vi "initGcode.vi"(6 "Che Do":bool=TRUE, 7 "gCode":T1, 8 "error in (no error)":errorcluster, 9 "PosSetG92":cluster{"X":dbl, "Y":dbl, "Z":dbl}, 10 "Gcode In":string, 11 "XuLyDataDisplay in":refnum<class "XuLyDataDisplay.lvclass">) -> (0 "error out":errorcluster, 2 "GcodeString Out":string, 3 "XuLyDataDisplay out":refnum<class "XuLyDataDisplay.lvclass">)   [LabVIEW 2017, in "LibraryGcode.lvlib" / "XuLyDataDisplay.lvclass"]
uses:
  XuLyDataDisplay.lvclass
  SelectGcode.ctl
  01552a10-2ba1-4855-bc3a-b1e10501afc1.vi
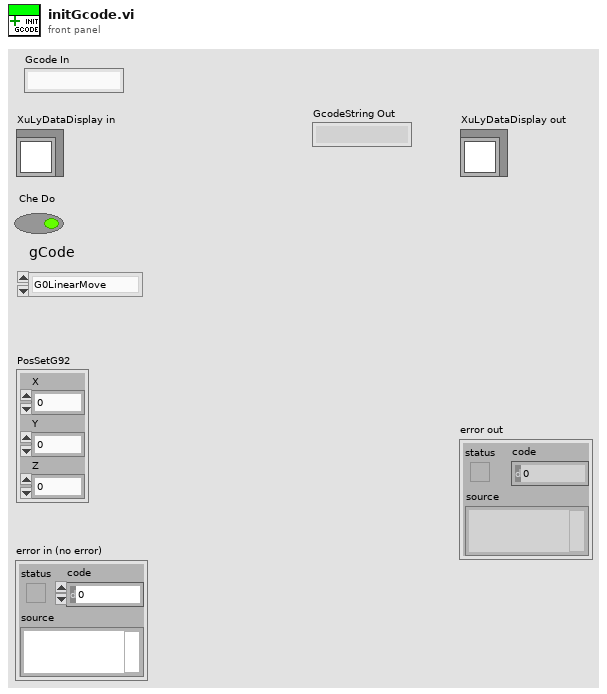
[diagram p1: front panel]
types:
  T1 = typedef "LibraryGcode.lvlib/XuLyDataDisplay.lvclass/SelectGcode.ctl" = enum16{"G0LinearMove", "G1XY", "G1LinearMove", "G2Arc", "G4Dwell", "G20InchUnit", "G21MilliUnit", "G28AutoHome", "G92SetPosition", "G90", "G91RelativePos", "JogX+", "JogX-", "JogY+", "JogY-", "JogZ+", "JogZ-", "sendGcodeString"}
  T2 = enum16{"Fan1", "Fan2", "Fan3", "PARA", "POS_DEGREE", "Solenoid", "Spindle", "TypeFirmware", "WaitPin", "MaxAcel", "MaxFeedrate", "MaxSize", "MaxStartAccel"}
  T3 = typedef "LibraryGcode.lvlib/TypeFirmwareControl.ctl" = enum16{"ScaraMarlin", "CncMarlin", "Mk4Due"}
  T4 = cluster{"PWM":dbl, "TypeFirmware":T3, "XYZ":cluster{"X":dbl, "Y":dbl, "Z":dbl}, "PARA":cluster{"STEP":i16, "FEEDRATE":dbl}, "DEGREES":cluster{"X":dbl, "Y":dbl}, "Solenoid":bool, "StartAccel":cluster{"P":dbl, "R":dbl, "T":dbl}}
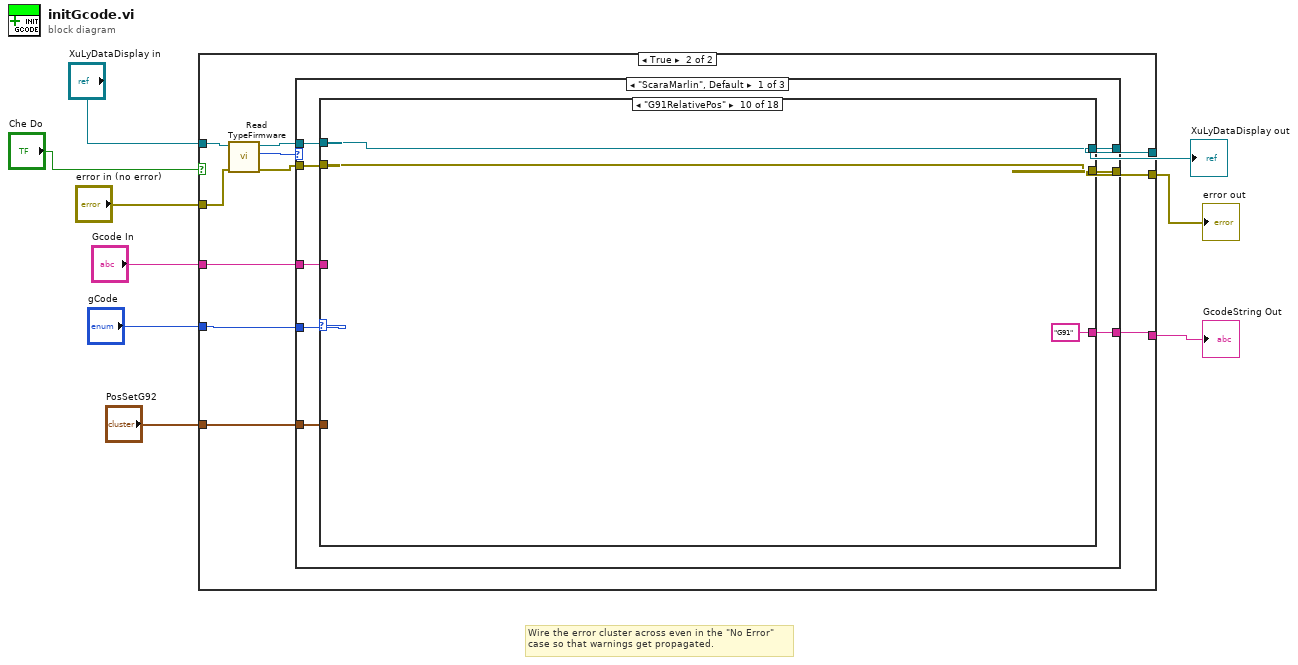
[diagram p0: block diagram]
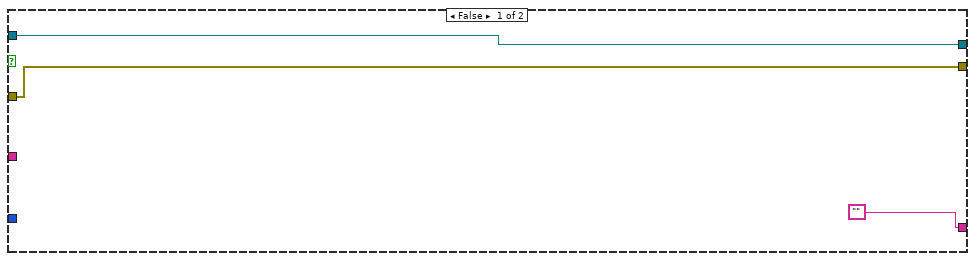
[diagram p2: hidden frame]
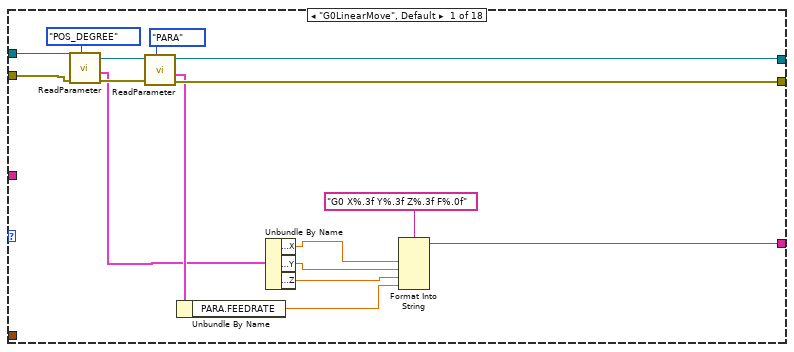
[diagram p3: hidden frame]
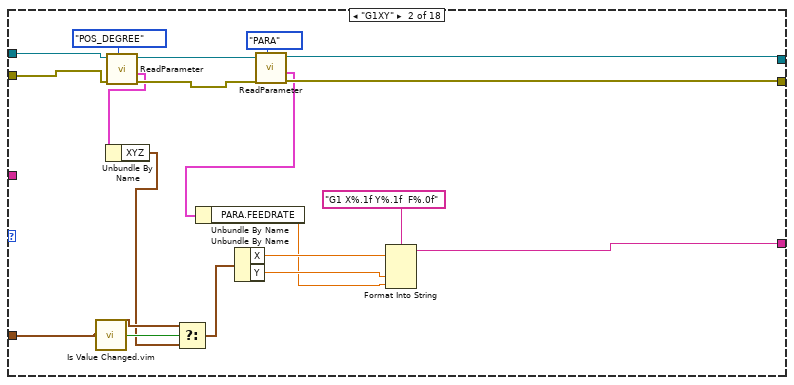
[diagram p4: hidden frame]
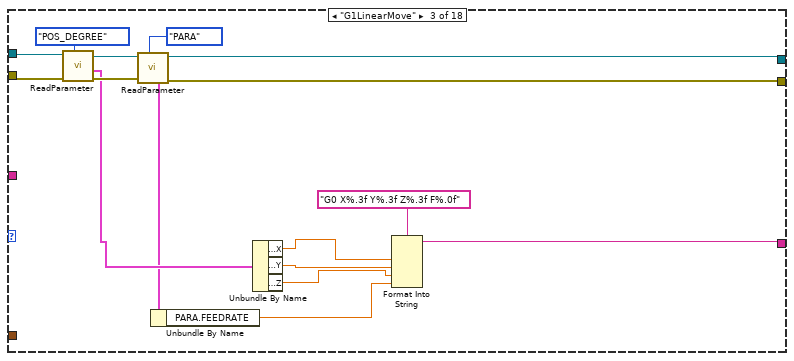
[diagram p5: hidden frame]
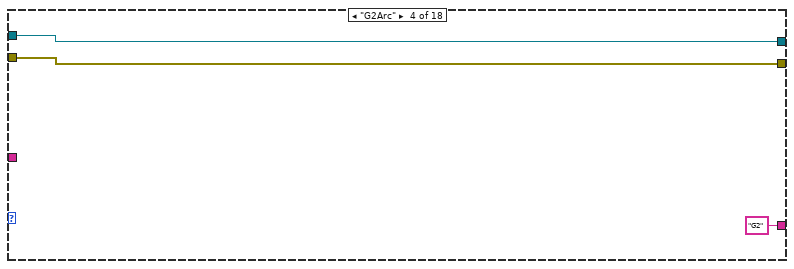
[diagram p6: hidden frame]
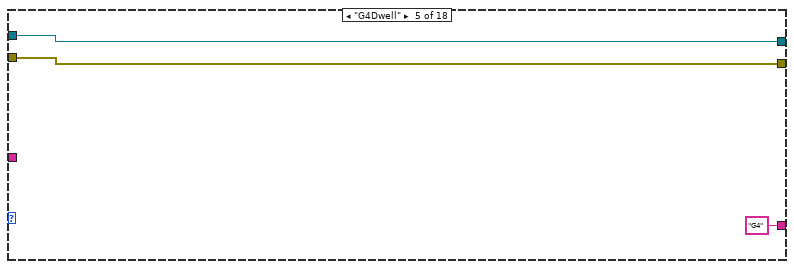
[diagram p7: hidden frame]
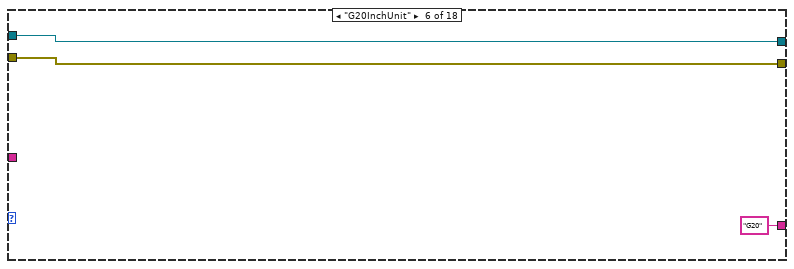
[diagram p8: hidden frame]
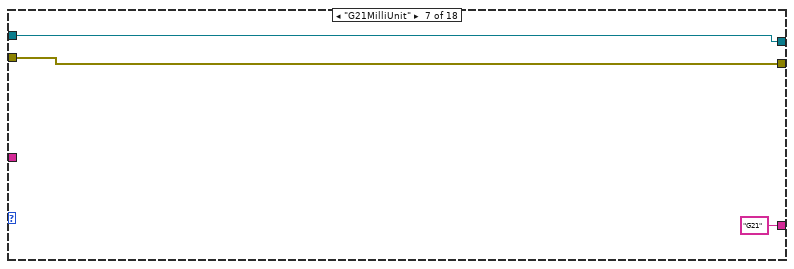
[diagram p9: hidden frame]
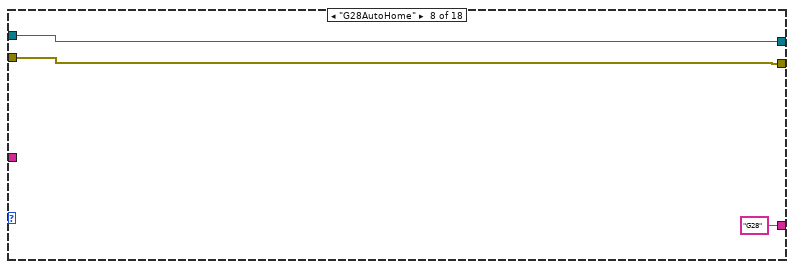
[diagram p10: hidden frame]
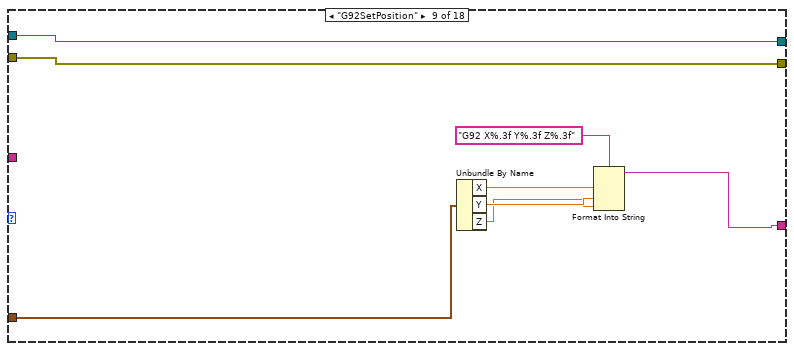
[diagram p11: hidden frame]
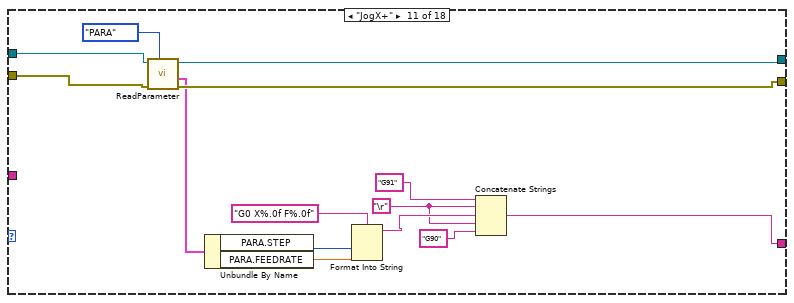
[diagram p12: hidden frame]
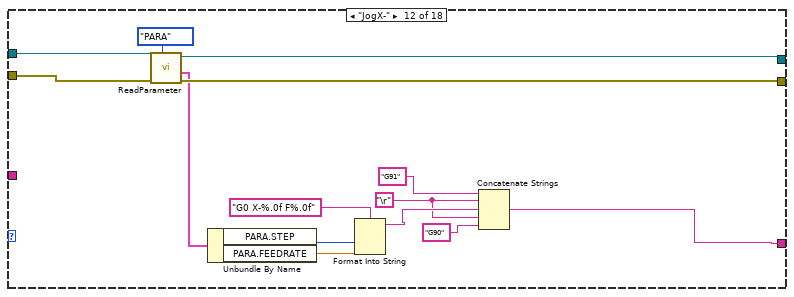
[diagram p13: hidden frame]
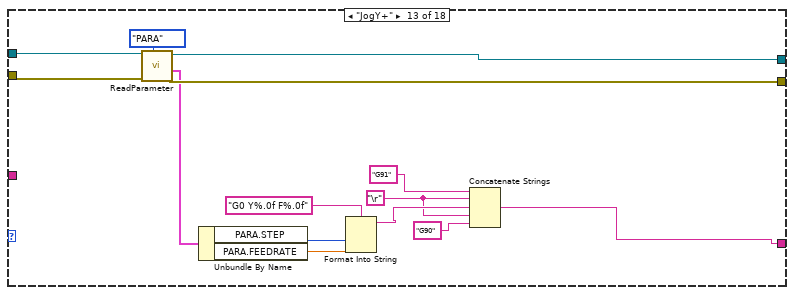
[diagram p14: hidden frame]
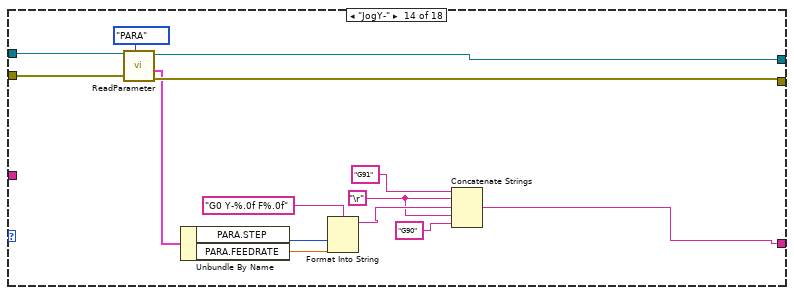
[diagram p15: hidden frame]
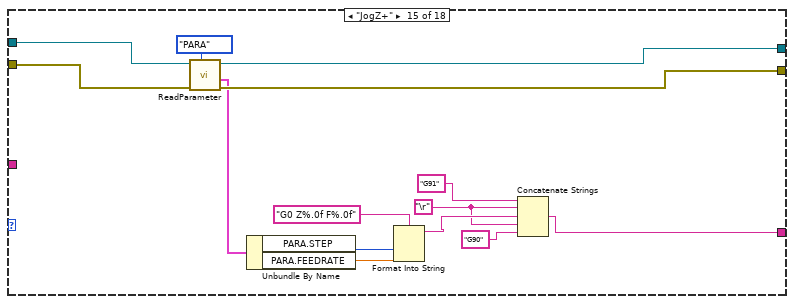
[diagram p16: hidden frame]
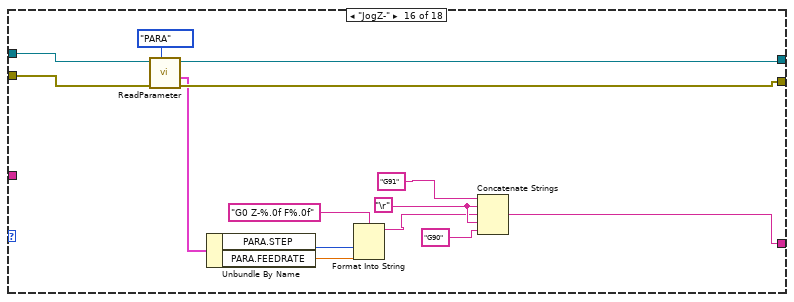
[diagram p17: hidden frame]
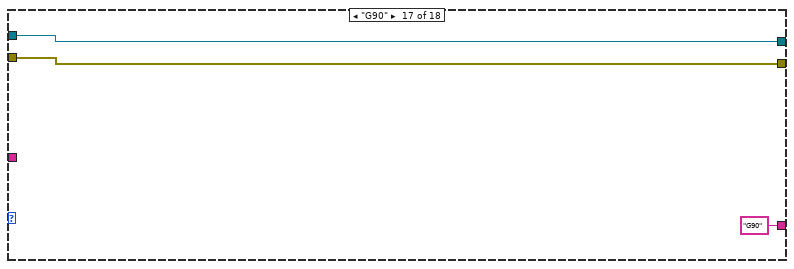
[diagram p18: hidden frame]
diagram:
  # "Wire the error cluster across even in the \"No Error\"\ncase so that warnings get propagated."
  n1 = case shown="True" "Che Do" {
    tunnel: [w11 w18] -> w9
    tunnel: [w12 w23] -> w8
    tunnel: "XuLyDataDisplay in" -> [w12 w21]
    tunnel: "gCode" -> [_ w17]
    tunnel: ["" w13] -> w5
    tunnel: "PosSetG92" -> [_ w16]
    tunnel: "error in (no error)" -> [w11 w15]
    tunnel: "Gcode In" -> [_ w14]
    frame False {
    }
    frame True {
      n2 = call-dynamic "Read TypeFirmware.vi"("error in (no error)"=w15, "ParameterConf in"=w21) -> ("error out"=w19:errorcluster, "TypeFirmware"=w20:T3, "ParameterConf out"=w22:refnum<class "XuLyDataDisplay.lvclass">)  [unwired: 7 in]
      n3 = case shown="\"ScaraMarlin\", Default" w20 {
        tunnel: [w28 w203 w209] -> w23
        tunnel: w22 -> [w27 w202 w209]
        tunnel: w19 -> [w29 w200 w208]
        tunnel: [w30 w201 w208] -> w18
        tunnel: w17 -> [w31 w199 _]
        tunnel: w16 -> [w26 _ _]
        tunnel: w14 -> [w24 _ _]
        tunnel: [w25 _ _] -> w13
        frame "ScaraMarlin", Default {
          n4 = case shown="\"G91RelativePos\"" w31 {
            tunnel: [w38 w59 w73 w83 w86 w89 w92 w95 w98 w106 w112 w126 w141 w154 w169 w181 w193 w196] -> w30
            tunnel: w29 -> [w40 w55 w74 w83 w86 w89 w92 w95 w98 w106 w114 w128 w140 w156 w168 w186 w193 w196]
            tunnel: [w37 w60 w72 w84 w87 w90 w93 w96 w99 w107 w113 w127 w142 w155 w170 w182 w194 w197] -> w28
            tunnel: w27 -> [w43 w56 w75 w84 w87 w90 w93 w96 w99 w107 w115 w129 w143 w157 w171 w187 w194 w197]
            tunnel: [w36 w63 w71 "G2" "G4" "G20" "G21" "G28" w101 "G91" w111 w125 w139 w153 w167 w183 "G90" w198] -> w25
            tunnel: w26 -> [_ w61 _ _ _ _ _ _ w100 _ _ _ _ _ _ _ _ _]
            tunnel: w24 -> [_ _ _ _ _ _ _ _ _ _ _ _ _ _ _ _ _ w198]
            frame "G0LinearMove", Default {
              n5 = call-dynamic "ReadParameter.vi"("ParameterConf in"=w43, "error in (no error)"=w40, "Parameter"=T2."POS_DEGREE") -> ("ParameterConf out"=w42:refnum<class "XuLyDataDisplay.lvclass">, "DataOutClust"=w32:T4, "error out"=w39:errorcluster)  [unwired: 4 in, 1 out]
              n6 = call-dynamic "ReadParameter.vi"("ParameterConf in"=w42, "error in (no error)"=w39, "Parameter"=T2."PARA") -> ("ParameterConf out"=w37:refnum<class "XuLyDataDisplay.lvclass">, "DataOutClust"=w33:T4, "error out"=w38:errorcluster)  [unwired: 4 in, 1 out]
              n7 = Unbundle By Name(w33) -> ("PARA.FEEDRATE"=w41:dbl)
              n8 = Unbundle By Name(w32) -> ("XYZ.X"=w46:dbl, "XYZ.Y"=w45:dbl, "XYZ.Z"=w44:dbl)
              n9 = Format Into String(format string="G0 X%.3f Y%.3f Z%.3f F%.0f", w46, w45, w44, w41) -> (resulting string=w36:string)  [unwired: 2 in, 1 out]
            }
            frame "G1XY" {
              n10 = call "Is Value Changed.vim"("value"=w61) -> ("changed or first call?"=w62:bool)
              n11 = call-dynamic "ReadParameter.vi"("ParameterConf in"=w56, "error in (no error)"=w55, "Parameter"=T2."POS_DEGREE") -> ("ParameterConf out"=w52:refnum<class "XuLyDataDisplay.lvclass">, "DataOutClust"=w50:T4, "error out"=w51:errorcluster)  [unwired: 4 in, 1 out]
              n12 = Unbundle By Name(w50) -> ("XYZ"=w49:cluster{"X":dbl, "Y":dbl, "Z":dbl})
              n13 = Select(t=w61, s=w62, f=w49) -> (s? t:f=w53:cluster{"X":dbl, "Y":dbl, "Z":dbl})
              n14 = Unbundle By Name(w53) -> ("X"=w65:dbl, "Y"=w64:dbl)
              n15 = call-dynamic "ReadParameter.vi"("ParameterConf in"=w52, "error in (no error)"=w51, "Parameter"=T2."PARA") -> ("ParameterConf out"=w60:refnum<class "XuLyDataDisplay.lvclass">, "DataOutClust"=w48:T4, "error out"=w59:errorcluster)  [unwired: 4 in, 1 out]
              n16 = Unbundle By Name(w48) -> ("PARA.FEEDRATE"=w57:dbl)
              n17 = Format Into String(format string="G1 X%.1f Y%.1f  F%.0f", w65, w64, w57) -> (resulting string=w63:string)  [unwired: 2 in, 1 out]
            }
            frame "G1LinearMove" {
              n18 = call-dynamic "ReadParameter.vi"("ParameterConf in"=w75, "error in (no error)"=w74, "Parameter"=T2."POS_DEGREE") -> ("ParameterConf out"=w78:refnum<class "XuLyDataDisplay.lvclass">, "DataOutClust"=w69:T4, "error out"=w76:errorcluster)  [unwired: 4 in, 1 out]
              n19 = call-dynamic "ReadParameter.vi"("ParameterConf in"=w78, "error in (no error)"=w76, "Parameter"=T2."PARA") -> ("ParameterConf out"=w72:refnum<class "XuLyDataDisplay.lvclass">, "DataOutClust"=w67:T4, "error out"=w73:errorcluster)  [unwired: 4 in, 1 out]
              n20 = Unbundle By Name(w67) -> ("PARA.FEEDRATE"=w77:dbl)
              n21 = Unbundle By Name(w69) -> ("XYZ.X"=w81:dbl, "XYZ.Y"=w80:dbl, "XYZ.Z"=w79:dbl)
              n22 = Format Into String(format string="G0 X%.3f Y%.3f Z%.3f F%.0f", w81, w80, w79, w77) -> (resulting string=w71:string)  [unwired: 2 in, 1 out]
            }
            frame "G2Arc" {
            }
            frame "G4Dwell" {
            }
            frame "G20InchUnit" {
            }
            frame "G21MilliUnit" {
            }
            frame "G28AutoHome" {
            }
            frame "G92SetPosition" {
              n23 = Unbundle By Name(w100) -> ("X"=w104:dbl, "Y"=w103:dbl, "Z"=w102:dbl)
              n24 = Format Into String(format string="G92 X%.3f Y%.3f Z%.3f", w104, w103, w102) -> (resulting string=w101:string)  [unwired: 2 in, 1 out]
            }
            frame "G91RelativePos" {
            }
            frame "JogX+" {
              w118 = "\r"
              n25 = call-dynamic "ReadParameter.vi"("ParameterConf in"=w115, "error in (no error)"=w114, "Parameter"=T2."PARA") -> ("ParameterConf out"=w113:refnum<class "XuLyDataDisplay.lvclass">, "DataOutClust"=w109:T4, "error out"=w112:errorcluster)  [unwired: 4 in, 1 out]
              n26 = Unbundle By Name(w109) -> ("PARA.STEP"=w121:i16, "PARA.FEEDRATE"=w120:dbl)
              n27 = Format Into String(format string="G0 X%.0f F%.0f", w121, w120) -> (resulting string=w122:string)  [unwired: 2 in, 1 out]
              n28 = Concatenate Strings("G91" ("string"), w118, w122, w118, "G90" ("string")) -> (w111:string)
            }
            frame "JogX-" {
              w132 = "\r"
              n29 = call-dynamic "ReadParameter.vi"("ParameterConf in"=w129, "error in (no error)"=w128, "Parameter"=T2."PARA") -> ("ParameterConf out"=w127:refnum<class "XuLyDataDisplay.lvclass">, "DataOutClust"=w124:T4, "error out"=w126:errorcluster)  [unwired: 4 in, 1 out]
              n30 = Unbundle By Name(w124) -> ("PARA.STEP"=w135:i16, "PARA.FEEDRATE"=w134:dbl)
              n31 = Format Into String(format string="G0 X-%.0f F%.0f", w135, w134) -> (resulting string=w136:string)  [unwired: 2 in, 1 out]
              n32 = Concatenate Strings("G91" ("string"), w132, w136, w132, "G90" ("string")) -> (w125:string)
            }
            frame "JogY+" {
              w146 = "\r"
              n33 = call-dynamic "ReadParameter.vi"("ParameterConf in"=w143, "error in (no error)"=w140, "Parameter"=T2."PARA") -> ("ParameterConf out"=w142:refnum<class "XuLyDataDisplay.lvclass">, "DataOutClust"=w138:T4, "error out"=w141:errorcluster)  [unwired: 4 in, 1 out]
              n34 = Unbundle By Name(w138) -> ("PARA.STEP"=w149:i16, "PARA.FEEDRATE"=w148:dbl)
              n35 = Format Into String(format string="G0 Y%.0f F%.0f", w149, w148) -> (resulting string=w150:string)  [unwired: 2 in, 1 out]
              n36 = Concatenate Strings("G91" ("string"), w146, w150, w146, "G90" ("string")) -> (w139:string)
            }
            frame "JogY-" {
              w160 = "\r"
              n37 = call-dynamic "ReadParameter.vi"("ParameterConf in"=w157, "error in (no error)"=w156, "Parameter"=T2."PARA") -> ("ParameterConf out"=w155:refnum<class "XuLyDataDisplay.lvclass">, "DataOutClust"=w152:T4, "error out"=w154:errorcluster)  [unwired: 4 in, 1 out]
              n38 = Unbundle By Name(w152) -> ("PARA.STEP"=w163:i16, "PARA.FEEDRATE"=w164:dbl)
              n39 = Format Into String(format string="G0 Y-%.0f F%.0f", w163, w164) -> (resulting string=w162:string)  [unwired: 2 in, 1 out]
              n40 = Concatenate Strings("G91" ("string"), w160, w162, w160, "G90" ("string")) -> (w153:string)
            }
            frame "JogZ+" {
              w174 = "\r"
              n41 = call-dynamic "ReadParameter.vi"("ParameterConf in"=w171, "error in (no error)"=w168, "Parameter"=T2."PARA") -> ("ParameterConf out"=w170:refnum<class "XuLyDataDisplay.lvclass">, "DataOutClust"=w166:T4, "error out"=w169:errorcluster)  [unwired: 4 in, 1 out]
              n42 = Unbundle By Name(w166) -> ("PARA.STEP"=w177:i16, "PARA.FEEDRATE"=w178:dbl)
              n43 = Format Into String(format string="G0 Z%.0f F%.0f", w177, w178) -> (resulting string=w176:string)  [unwired: 2 in, 1 out]
              n44 = Concatenate Strings("G91" ("string"), w174, w176, w174, "G90" ("string")) -> (w167:string)
            }
            frame "JogZ-" {
              w192 = "\r"
              n45 = call-dynamic "ReadParameter.vi"("ParameterConf in"=w187, "error in (no error)"=w186, "Parameter"=T2."PARA") -> ("ParameterConf out"=w182:refnum<class "XuLyDataDisplay.lvclass">, "DataOutClust"=w180:T4, "error out"=w181:errorcluster)  [unwired: 4 in, 1 out]
              n46 = Unbundle By Name(w180) -> ("PARA.STEP"=w185:i16, "PARA.FEEDRATE"=w184:dbl)
              n47 = Format Into String(format string="G0 Z-%.0f F%.0f", w185, w184) -> (resulting string=w188:string)  [unwired: 2 in, 1 out]
              n48 = Concatenate Strings("G91" ("string"), w192, w188, w192, "G90" ("string")) -> (w183:string)
            }
            frame "G90" {
            }
            frame "sendGcodeString" {
            }
          }
        }
        frame "CncMarlin" {
          n49 = case shown="\"G1XY\"" w199 {
            tunnel: [w205 w207] -> w203
            tunnel: w202 -> [w205 w207]
            tunnel: [w204 w206] -> w201
            tunnel: w200 -> [w204 w206]
            frame "G0LinearMove", Default {
            }
            frame "G1XY" {
            }
          }
        }
        frame "Mk4Due" {
        }
      }
    }
  }
  "error out" <- w9
  "XuLyDataDisplay out" <- w8
  "GcodeString Out" <- w5
